vi "read_params.vi"(8 "error in (no error)":errorcluster, 11 "RANSACRegressor in":refnum<class "RANSACRegressor.lvclass">) -> (0 "error out":errorcluster, 2 "params":T1={"base_estimator"="None", "min_samples"={"min_samples_type"="None", "min_samples_int"=1, "min_samples_float"=0.1}, "residual_threshold"={"residual_threshold_float"=0.0, "residual_threshold_type"="None"}, "max_trials"=100.0, "max_skips"=18446744073709551615, "stop_n_inliers"=18446744073709551615, "stop_score"=1.8446744073709552e+19, "stop_probability"=0.99, "loss"="absolute_loss", "random_state"=0.0}, 3 "RANSACRegressor out":refnum<class "RANSACRegressor.lvclass">)   [LabVIEW 2020, in "RANSACRegressor.lvclass"]
uses:
  RANSACRegressor.lvclass
  Controls/ransac_regressor_params.ctl
  RANSACRegressor.lvclass/RANSACRegressor.ctl
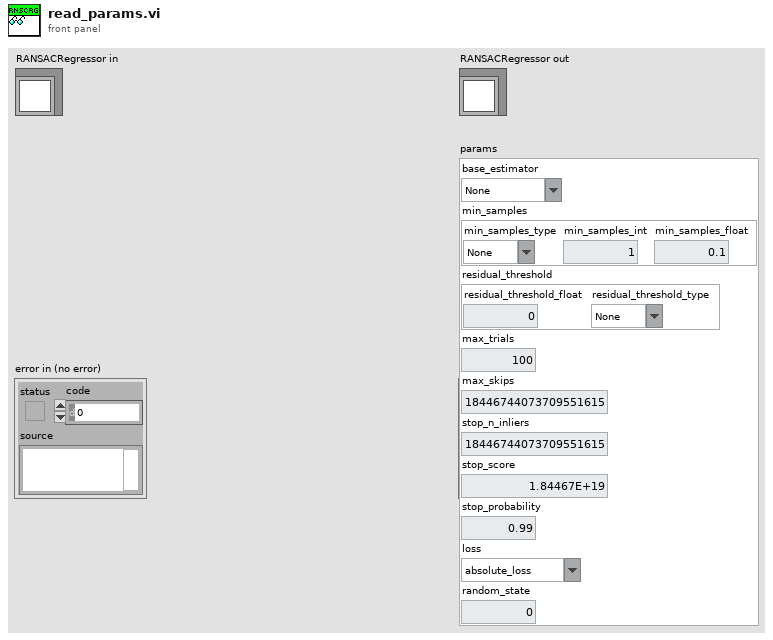
[diagram p1: front panel]
types:
  T1 = typedef "ransac_regressor_params.ctl" = cluster{"base_estimator":string, "min_samples":cluster{"min_samples_type":string, "min_samples_int":i32, "min_samples_float":dbl}, "residual_threshold":cluster{"residual_threshold_float":dbl, "residual_threshold_type":string}, "max_trials":dbl, "max_skips":u64, "stop_n_inliers":u64, "stop_score":dbl, "stop_probability":dbl, "loss":string, "random_state":dbl}
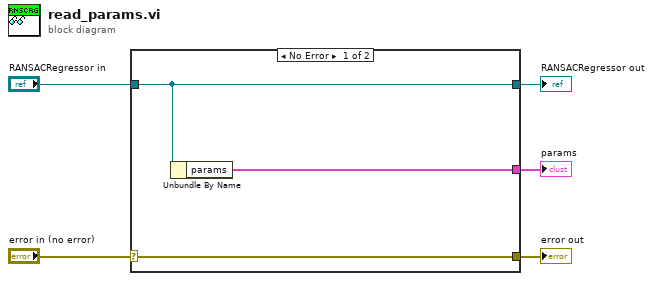
[diagram p0: block diagram]
diagram:
  n1 = case shown="No Error" "error in (no error)" {
    selector: "error in (no error)" -> [w8 w9]
    tunnel: [w8 w9] -> w4
    tunnel: [w7 w10] -> w2
    tunnel: "RANSACRegressor in" -> [w7 w10]
    tunnel: [w6 _] -> w1
    frame No Error {
      n2 = Unbundle By Name(w7) -> ("params"=w6:T1)
    }
    frame Error {
    }
  }
  "error out" <- w4
  "RANSACRegressor out" <- w2
  "params" <- w1
